vi "PH_PILS.PC _Enabling MainAmp changed.vi"(0 "i ref in":refnum<vi>, 5 "error in":errorcluster) -> (14 "i ref out":refnum<vi>, 19 "error out":errorcluster)   [LabVIEW 2014, in "PH_PILS.lvlib"]
uses:
  PH_PILS.lvlib
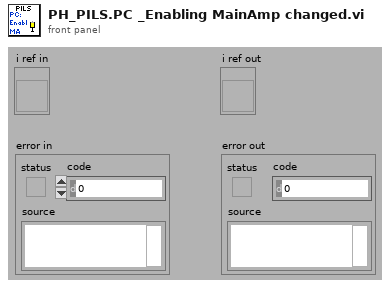
[diagram p1: front panel]
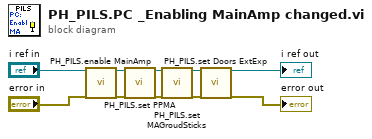
[diagram p0: block diagram]
diagram:
  n1 = call "PH_PILS.enable MainAmp.vi"("i ref in"="i ref in", "error in"="error in") -> ("i ref out"=w3:refnum<vi>, "error out"=w5:errorcluster)  [unwired: 16 in]
  n2 = call "PH_PILS.set PPMA.vi"("i ref in"=w3, "error in"=w5) -> ("i ref out"=w4:refnum<vi>, "error out"=w6:errorcluster)  [unwired: 16 in]
  n3 = call "PH_PILS.set MAGroudSticks.vi"("i ref in"=w4, "error in"=w6) -> ("i ref out"=w7:refnum<vi>, "error out"=w9:errorcluster)  [unwired: 16 in]
  n4 = call "PH_PILS.set Doors ExtExp.vi"("i ref in"=w7, "error in"=w9) -> ("i ref out"=→"i ref out":refnum<vi>, "error out"=→"error out":errorcluster)  [unwired: 16 in]
